vi "task2.vi"() -> ()   [LabVIEW 2021]
uses:
  <vilib>/Utility/file.llb/Write Delimited Spreadsheet (DBL).vi
panel:
  out "Array":dbl[](array[numeric])
  in  "Numeric":i32
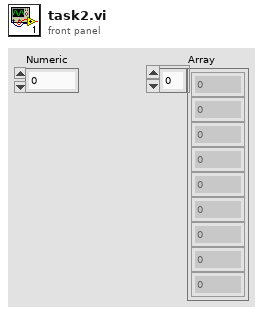
[diagram p1: front panel]
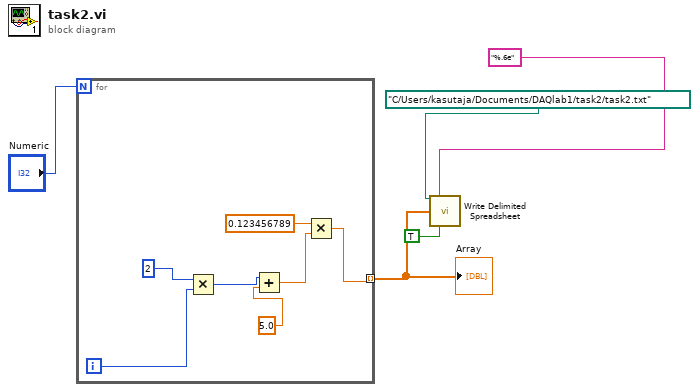
[diagram p0: block diagram]
diagram:
  n1 = for {
    N: "Numeric" -> [_]
    tunnel: [w6] -> w4 mode=indexing
    i -> [w11]
    n2 = Multiply(x=2, y=w11) -> (x*y=w9:i32)
    n3 = Add(x=w9, y=5.0 ("x*y")) -> (x+y=w7:dbl)
    n4 = Multiply(x=0.123456789, y=w7) -> (x*y=w6:dbl)
  }
  "Array" <- w4
  n5 = call-poly <vilib>:"Write Delimited Spreadsheet.vi"("file path (dialog if empty)"=path "C:/Users/kasutaja/Documents/DAQlab1/task2/task2.txt" ("Path"), "format (%.3f)"="%.6e", "1D data"=w4, "transpose? (no:F)"=TRUE) -> ()  [unwired: 10 in, 2 out]
